vi "Write User Event with Error Support.vi"(6 "優先度（通常）":T1, 7 "EvCmd":string, 8 "エラー入力（エラーなし）":errorcluster, 10 "データ":variant, 11 "ユーザイベント入力":refnum<user-event>) -> (0 "エラー出力":errorcluster, 3 "ユーザイベント出力":refnum<user-event>)   [LabVIEW 2014]
uses:
  Ctl/Event Cluster.ctl
  <vilib>/event_ctls.llb/usereventprio.ctl
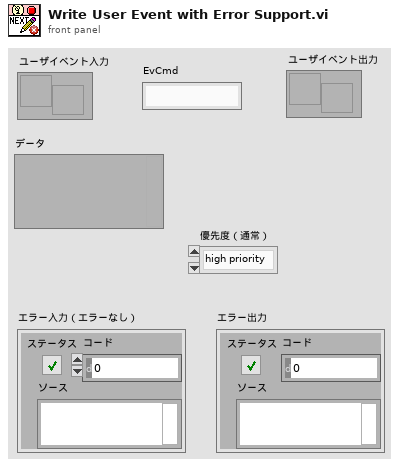
[diagram p1: front panel]
types:
  T1 = typedef "usereventprio.ctl" = enum32{"high priority", "normal priority"}
  T2 = typedef "Event Cluster.ctl" = cluster{"コマンド":string, "バリアント":variant}
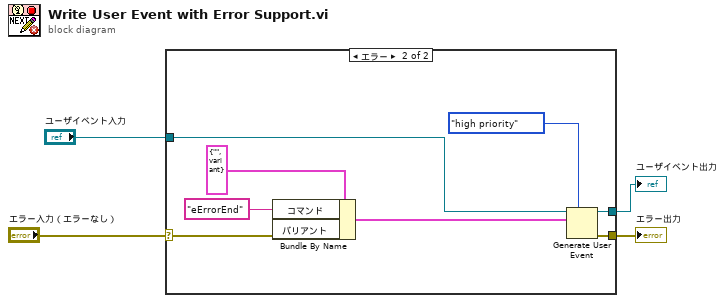
[diagram p0: block diagram]
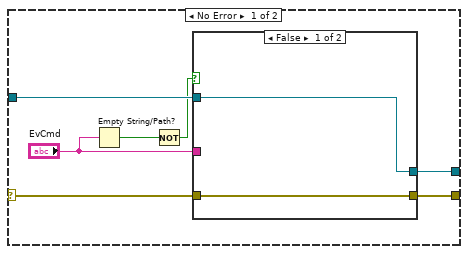
[diagram p2: hidden frame]
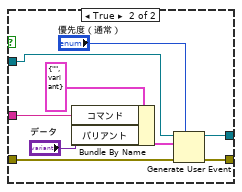
[diagram p3: hidden frame]
diagram:
  n1 = case shown="エラー" "エラー入力（エラーなし）" {
    selector: "エラー入力（エラーなし）" -> [w8 w24]
    tunnel: [w11 w29] -> w4
    tunnel: [w10 w28] -> w3
    tunnel: "ユーザイベント入力" -> [w9 w30]
    frame No Error {
      n2 = Empty String/Path?(string/path="EvCmd") -> (empty?=w6:bool)
      n3 = Not(x=w6) -> (.not. x?=w5:bool)
      n4 = case shown="FALSE" w5 {
        tunnel: [w13 w21] -> w11
        tunnel: [w12 w20] -> w10
        tunnel: w9 -> [w12 w19]
        tunnel: w8 -> [w13 w16]
        tunnel: "EvCmd" -> [_ w15]
        frame False {
        }
        frame True {
          n5 = Bundle By Name(cluster=T2 {"コマンド"="", "バリアント"=variant} ("Event Cluster"), "コマンド"=w15, "バリアント"="データ") -> (w22:T2)
          n6 = Generate User Event(priority (normal)="優先度（通常）", user event=w19, event data cluster=w22, error in=w16) -> (user event out=w20:refnum<user-event>, error out=w21:errorcluster)
        }
      }
    }
    frame Error {
      n7 = Bundle By Name(cluster=T2 {"コマンド"="", "バリアント"=variant} ("Event Cluster"), "コマンド"="eErrorEnd", "バリアント"=w24) -> (w23:T2)
      n8 = Generate User Event(priority (normal)=usereventprio."high priority" ("優先度（通常）"), user event=w30, event data cluster=w23) -> (user event out=w28:refnum<user-event>, error out=w29:errorcluster)  [unwired: 1 in]
    }
  }
  "エラー出力" <- w4
  "ユーザイベント出力" <- w3
